vi "coord trans.vi"(1 "x":dbl[](array[numeric]), 2 "Offset":dbl[](array[numeric]), 3 "A":T1) -> (0 "dgemv":dbl[](array[numeric]))   [LabVIEW 2017]
uses:
  <vilib>/Analysis/Matrix/Datatypes/RealMatrix.ctl
  <vilib>/Analysis/BLAS.llb/dgemv - General Matrix-Vector Product (DBL).vi
  <vilib>/Analysis/NI_AALBLAS.lvlib
  <vilib>/Analysis/Matrix/NI_Matrix.lvlib
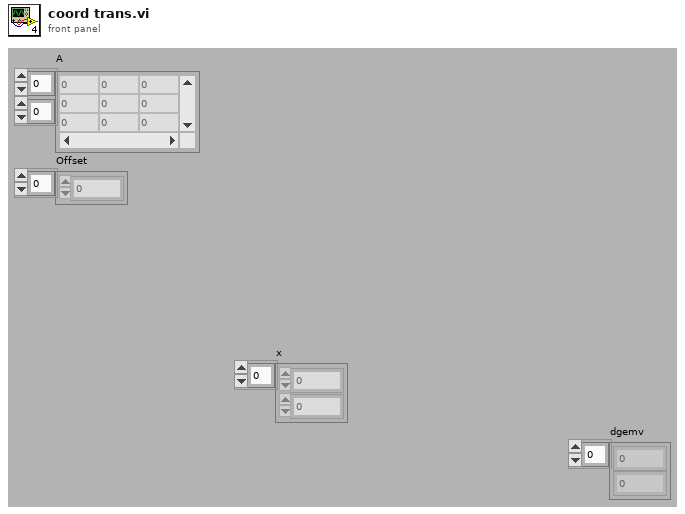
[diagram p1: front panel]
types:
  T1 = typedef "NI_Matrix.lvlib/RealMatrix.ctl" = dbl[][]
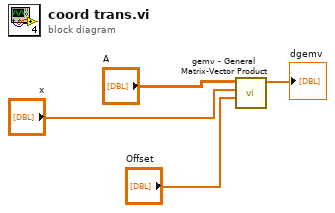
[diagram p0: block diagram]
diagram:
  n1 = call-poly <vilib>:"gemv - General Matrix-Vector Product.vi"("y"="Offset", "x"="x", "A"="A") -> ("dgemv"=→"dgemv":dbl[])  [unwired: 7 in, 1 out]
